vi "Pace Impulse.vi"(1 "P-Waves Locations (s)":dbl[](array[numeric]) format="%.2p", 2 "R-Wave Locations (s)":dbl[](array[numeric]) format="%.2p", 3 "ECG Data":dbl[](array[numeric])) -> (0 "Impulses":waveform(dbl)(graph))   [LabVIEW 2018]
uses:
  <vilib>/Analysis/NI_AALBase.lvlib
panel:
  out "Init":dbl[](array[numeric]) format="%.2p"
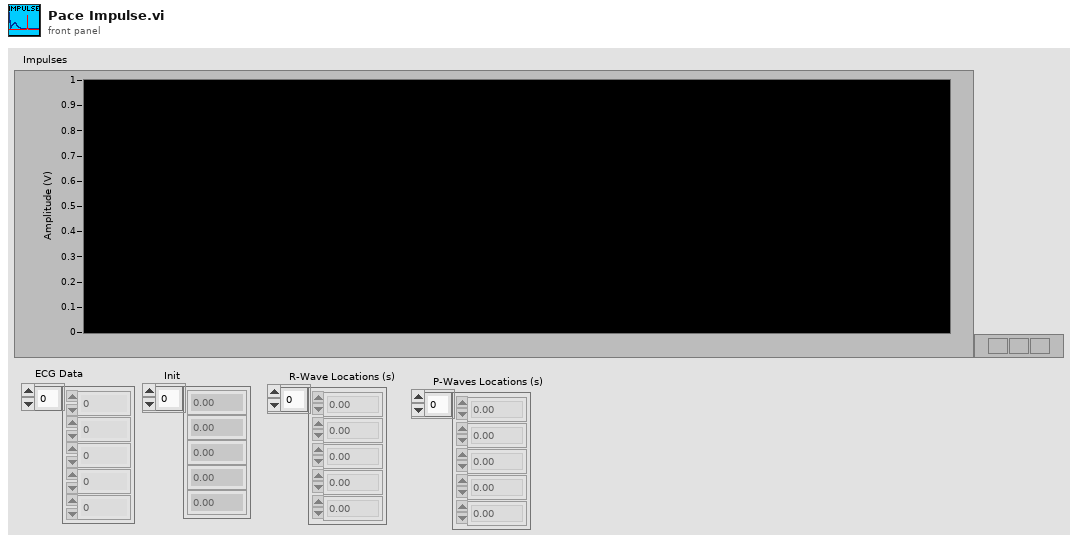
[diagram p1: front panel]
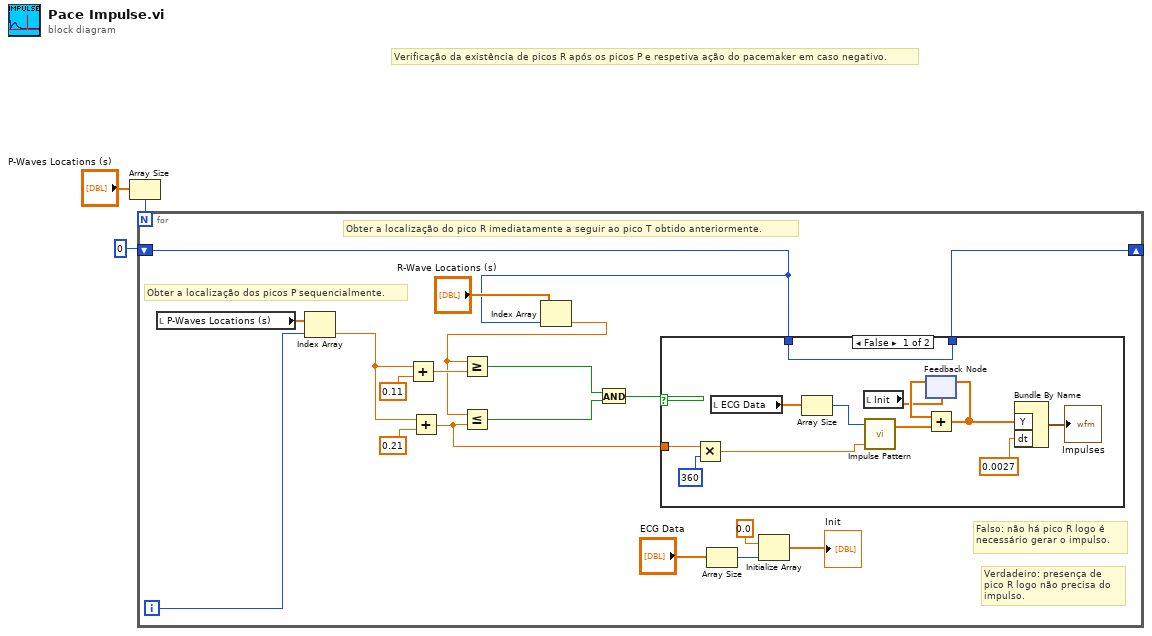
[diagram p0: block diagram]
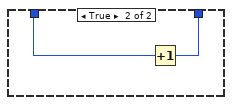
[diagram p2: hidden frame]
diagram:
  # "Verificação da existência de picos R após os picos P e respetiva ação do pacemaker em caso negativo."
  n1 = Array Size(array="P-Waves Locations (s)") -> (size(s)=w3:i32)
  n2 = for {
    N: w3 -> [_]
    shift-right: [w5] -> _
    shift-left: 0 -> [w4]
    i -> [w9]
    # "Verdadeiro: presença de pico R logo não precisa do impulso."
    # "Falso: não há pico R logo é necessário gerar o impulso."
    # "Obter a localização dos picos P sequencialmente."
    # "Obter a localização do pico R imediatamente a seguir ao pico T obtido anteriormente."
    n3 = local read "P-Waves Locations (s)"() -> (w14:dbl[])
    n4 = Index Array(array=w14, index=w9) -> (element=w20:dbl)
    n5 = Add(x=w20, y=0.11) -> (x+y=w21:dbl)
    n6 = Add(x=w20, y=0.21) -> (x+y=w11:dbl)
    n7 = Index Array(array="R-Wave Locations (s)", index=w4) -> (element=w6:dbl)
    n8 = Greater Or Equal?(x=w6, y=w21) -> (x >= y?=w19:bool)
    n9 = Less Or Equal?(x=w6, y=w11) -> (x <= y?=w18:bool)
    n10 = And(x=w19, y=w18) -> (x .and. y?=w15:bool)
    n11 = case shown="False" w15 {
      tunnel: [w22 w35] -> w5
      tunnel: w4 -> [w22 w34]
      tunnel: w11 -> [w24 _]
      frame False {
        n12 = Multiply(x=w24, y=360 ("width")) -> (x*y=w26:dbl)
        n13 = local read "ECG Data"() -> (w29:dbl[])
        n14 = Array Size(array=w29) -> (size(s)=w28:i32)
        n15 = local read "Init"() -> (w23:dbl[])
        n16 = call <vilib>:"Impulse Pattern.vi"("delay"=w26, "samples"=w28) -> ("Impulse Pattern"=w27:dbl[])  [unwired: 1 in, 1 out]
        n17 = feedback #1(w23) -> (w33:dbl[])
        n18 = Add(x=w33, y=w27) -> (x+y=w31:dbl[])
        n19 = feedback-in #1(w31) -> ()
        n20 = Bundle By Name ("Build Waveform")("Y"=w31, "dt"=0.0027) -> (→"Impulses":waveform(dbl))  [unwired: 1 in]
      }
      frame True {
        n21 = Increment(x=w34) -> (x+1=w35:i32)
      }
    }
    n22 = Array Size(array="ECG Data") -> (size(s)=w17:i32)
    n23 = Initialize Array(0.0 ("element"), w17) -> (→"Init":dbl[])
  }
